vi "CSMinfo.vi"(4 "Error In":errorcluster, 7 "Command":string) -> (0 "Error Out":errorcluster, 3 "Response":string)   [LabVIEW 2018]
uses:
  MOKO_LabViewLibrary/MokoLowLevel/MokoLowLovelControl/MLLC_Mode.ctl
  data/CSMinfo.ctl
panel:
  in  "Utility name":string="CSMinfo"
  in  "Error Code":i32=5475
  in  "Settings":T2={"Saved Data"=variant, "Permanent data"={"Общие сведения"={"Регистрационный номер заказа"="", "Идентификация (шифр) образца"="", "IMEI образца"="", "НД, устанавливающий требования"="", "Методы испытаний (измерений)"="", "Дата начала испытаний"="", "Дата завершения испытаний"=""}, "Климатические условия внешней среды"={"Температура окружающего воздуха"="", "Относительная влажность воздуха"="", "Атмосферное давление"=""}, "Окно с настройками"={"Режим звонка связь"=0, "Напряжение источника"=0, "Условия окружающей среды"=0, "Номер образца"=0, "Источник питания"=0, "Номер испытания"=0, "Режим звонка тональный модем"=0, "Количество итераций TM"=100.0, "Аутентификация"=0, "Колличество повторов измерений"=1.0, "Сим карта"=0, "VISA adress of CMW500"="", "Input attenuation"=1.0, "Output attenuation"=1.0, "Call Release Type"=0, "GSM Band"=0, "BCCH Channel Number"=0.0, "TCH Channel Number"=0.0, "Codec"=0, "AWGN"=0, "snrRatioInDb"=0.0, "GSM Fading"=0, "UL C/I ratio"=0, "Use a custom network ID"=FALSE, "MCC (Mobile Country Code)"=0.0, "MNC (Mobile Network Code)"=0.0, "NCC (Network Color Code)"=0.0, "MNC digit count"=0, "BCC (Base station Color Code)"=0.0, "LAC (Location Area Code)"=0.0, "RAC (Routing Area Code)"=0.0, "Cell Identity"=0.0, "Override UE ID"=FALSE, "MCC (UE Mobile Country Code)"=0.0, "MNC (UE Mobile Network Code)"=0.0, "MSIN (Mobile Subscription ID)"=0.0, "InputScaleFactor"=0, "OutputScaleFactor"=0, "Post MSD wave file playback 3GPP  26.269 \nEU_DTMF_tones"=FALSE, "Scenario"=0, "AlAckBehavior"=0, "PSAP listens for PUSH"=FALSE, "BCCH Channel Power"=0.0, "TCH Channel Power"=0.0, "Setting Path"=path "", "Алгоритм дозвона"=0}}} {"Permanent data"."Окно с настройками"."Алгоритм дозвона" items=["Standart", "Recall"]; "Permanent data"."Окно с настройками"."AlAckBehavior" items=["POSITIVE", "CLEAR_DOWN", "LOOP_BACK_MSD_PART"]; "Permanent data"."Окно с настройками"."Scenario" items=["NORMAL", "NORMAL_IMMEDIATE_START", "TIMEOUT_T3", "ALLRV_REQ", "SUPPRESS_MSD", "SUPPRESS_ALACK", "SUPPRESS_SEND_MSD"]; "Permanent data"."Окно с настройками"."OutputScaleFactor" items=["ONE", "QUARTER", "HALF", "TWO", "FOUR"]; "Permanent data"."Окно с настройками"."InputScaleFactor" items=["ONE", "QUARTER", "HALF", "TWO", "FOUR"]; "Permanent data"."Окно с настройками"."MNC digit count" items=["TWO", "THREE"]; "Permanent data"."Окно с настройками"."UL C/I ratio" items=["Ci1Db", "Ci4Db", "Ci7Db", "Ci10Db", "Ci13Db", "Ci16Db"]; "Permanent data"."Окно с настройками"."GSM Fading" items=["GsmFadingOff", "GsmEtsiTs103412DlFading", "GsmEtsiTs103412UlFading", "GsmEtsiTs103412DlUlFading"]; "Permanent data"."Окно с настройками"."AWGN" items=["Off", "50MhzAwgn"]; "Permanent data"."Окно с настройками"."Codec" items=["FRV2", "AMRH_GMSK_7K95", "AMRH_GMSK_7K40", "AMRH_GMSK_6K70", "AMRH_GMSK_5K90", "AMRH_GMSK_5K15", "AMRH_GMSK_4K75", "AMRF_GMSK_12K20", "AMRF_GMSK_10K20", "AMRF_GMSK_7K95", "AMRF_GMSK_7K40 ", "AMRF_GMSK_6K70", "AMRF_GMSK_5K90", "AMRF_GMSK_5K15", "AMRF_GMSK_4K75", "FRV1", "HRV1", "WAMR_GMSK_6K60", "WAMR_GMSK_8K85", "WAMR_GMSK_12K65"]; "Permanent data"."Окно с настройками"."GSM Band" items=["GSM450", "GSM850", "GSM900", "GSM1800", "GSM1900"]; "Permanent data"."Окно с настройками"."Call Release Type" items=["NormalRelease", "CallInterruption"]; "Permanent data"."Окно с настройками"."Сим карта" items=["SIM", "eSIM"]; "Permanent data"."Окно с настройками"."Колличество повторов измерений" min=1.0 max=100.0 format="%#_3g"; "Permanent data"."Окно с настройками"."Аутентификация" items=["On", "Off"]; "Permanent data"."Окно с настройками"."Режим звонка тональный модем" items=["Автоматически (AT) GEMALTO", "Автоматически (AT) SIMCOM", "Автоматически (AT) SIMCOM SIM7600E-H", "Автоматически (AT) TELIT", "Автоматически (AT) PROGRESS", "Автоматически (AT) PROGRESS GREEN", "Автоматически (AT) PROGRESS BLUE", "Автоматически (реле)", "Вручную"]; "Permanent data"."Окно с настройками"."Номер испытания" items=["1", "2", "3"]; "Permanent data"."Окно с настройками"."Источник питания" items=["Не используется", "IT6332A"]; "Permanent data"."Окно с настройками"."Номер образца" items=["1", "2", "3"]; "Permanent data"."Окно с настройками"."Условия окружающей среды" items=["UnormTnorm", "UminTmin", "UmaxTmin", "UminTmax", "UmaxTmax", "TypeA", "TypeB"]; "Permanent data"."Окно с настройками"."Напряжение источника" items=["12", "24"]; "Permanent data"."Окно с настройками"."Режим звонка связь" items=["Автоматически (AT) GEMALTO", "Автоматически (AT) SIMCOM", "Автоматически (AT) SIMCOM SIM7600E-H", "Автоматически (AT) TELIT", "Автоматически (AT) PROGRESS", "Автоматически (AT) PROGRESS GREEN", "Автоматически (AT) PROGRESS BLUE", "Автоматически (реле)", "Вручную"]}
  in  "Mode":T3=enum."Check"
  # "CSMinfo"
  # "Default Settings"
  # "1. Общие настройки"
  # "Настройки модема по умолчанию"
  # "CMW500"
  # "PSAP"
  # "8.6.6"
  # "8.6.7"
  # "GSM"
  # "2. Настройки связи"
  # "8.6.8 (Use parameter NORMAL_IMMEDIATE_START)"
  # "8.6.9 (Use parameter LOOP_BACK_MSD_PART)"
  # "8.6.6"
  # "3. Настройки тонального модема"
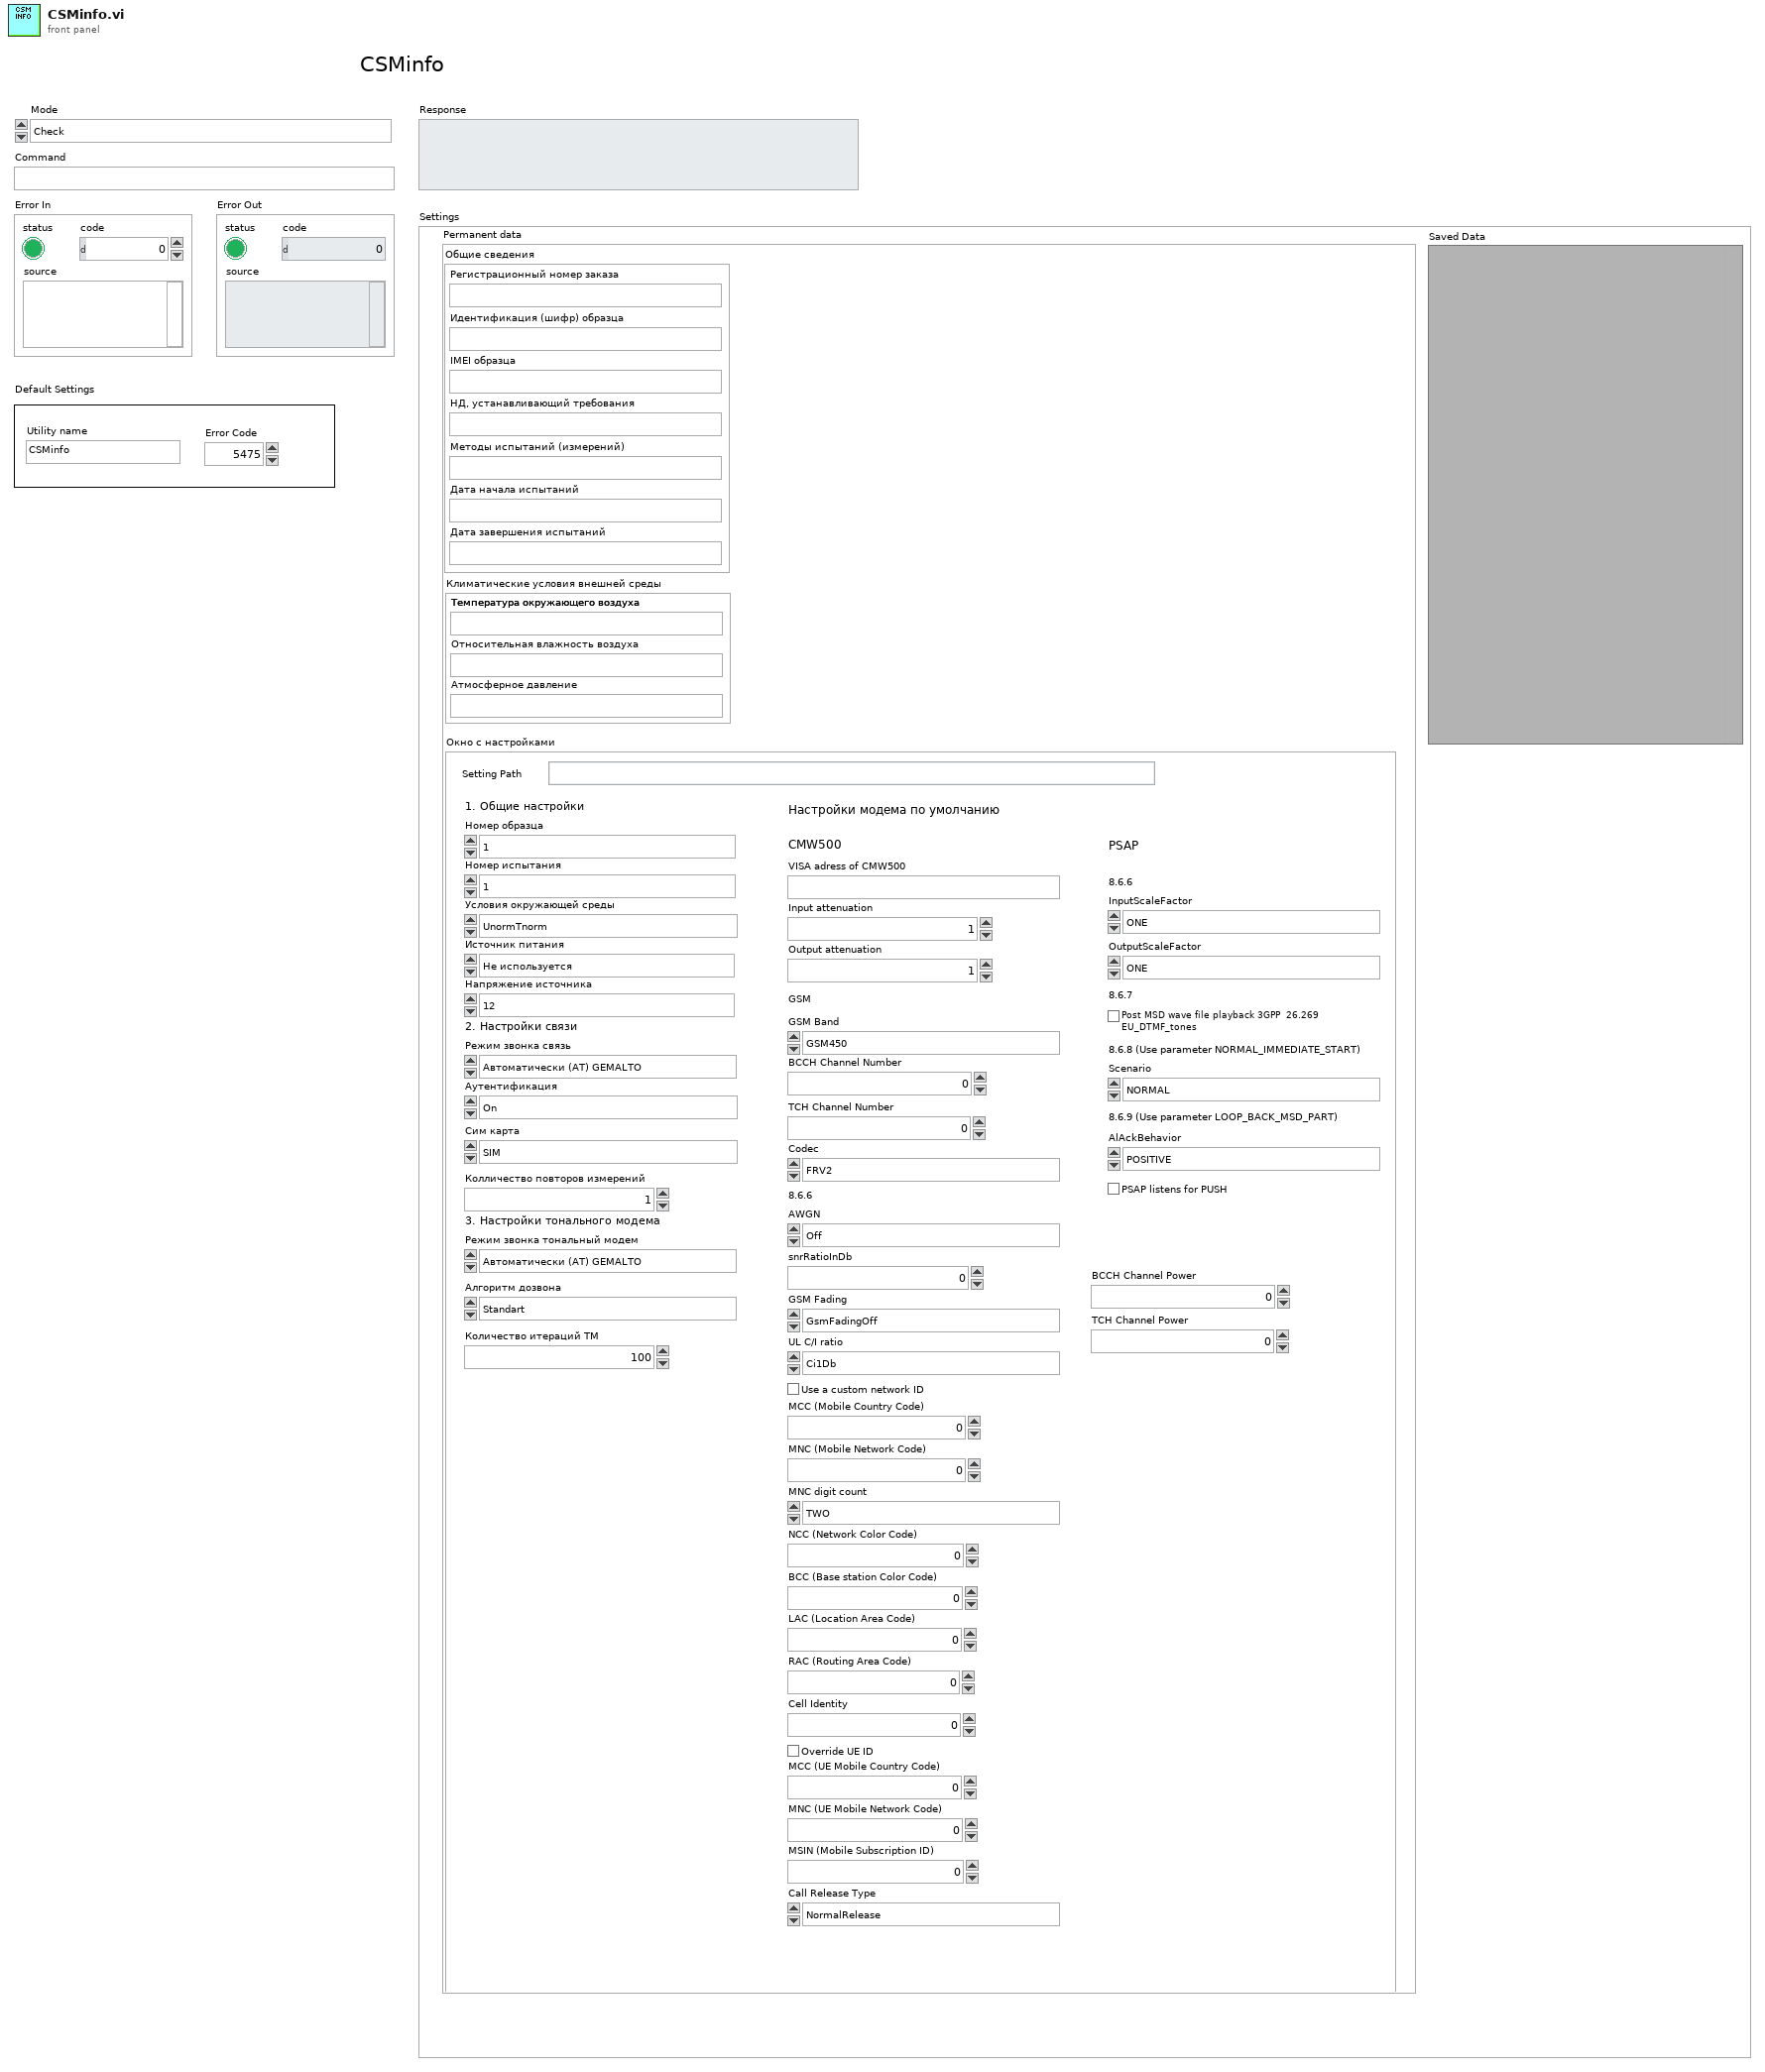
[diagram p1: front panel]
types:
  T1 = typedef "CSMinfo.ctl" = cluster{"Общие сведения":cluster{"Регистрационный номер заказа":string, "Идентификация (шифр) образца":string, "IMEI образца":string, "НД, устанавливающий требования":string, "Методы испытаний (измерений)":string, "Дата начала испытаний":string, "Дата завершения испытаний":string}, "Климатические условия внешней среды":cluster{"Температура окружающего воздуха":string, "Относительная влажность воздуха":string, "Атмосферное давление":string}, "Окно с настройками":cluster{"Режим звонка связь":u16, "Напряжение источника":u16, "Условия окружающей среды":u16, "Номер образца":u16, "Источник питания":u16, "Номер испытания":u16, "Режим звонка тональный модем":u16, "Количество итераций TM":dbl, "Аутентификация":u16, "Колличество повторов измерений":dbl, "Сим карта":u16, "VISA adress of CMW500":string, "Input attenuation":dbl, "Output attenuation":dbl, "Call Release Type":u16, "GSM Band":u16, "BCCH Channel Number":dbl, "TCH Channel Number":dbl, "Codec":u16, "AWGN":u16, "snrRatioInDb":dbl, "GSM Fading":u16, "UL C/I ratio":u16, "Use a custom network ID":bool, "MCC (Mobile Country Code)":dbl, "MNC (Mobile Network Code)":dbl, "NCC (Network Color Code)":dbl, "MNC digit count":u16, "BCC (Base station Color Code)":dbl, "LAC (Location Area Code)":dbl, "RAC (Routing Area Code)":dbl, "Cell Identity":dbl, "Override UE ID":bool, "MCC (UE Mobile Country Code)":dbl, "MNC (UE Mobile Network Code)":dbl, "MSIN (Mobile Subscription ID)":dbl, "InputScaleFactor":u16, "OutputScaleFactor":u16, "Post MSD wave file playback 3GPP  26.269 \nEU_DTMF_tones":bool, "Scenario":u16, "AlAckBehavior":u16, "PSAP listens for PUSH":bool, "BCCH Channel Power":dbl, "TCH Channel Power":dbl, "Setting Path":path, "Алгоритм дозвона":u16}}
  T2 = cluster{"Saved Data":variant, "Permanent data":T1}
  T3 = typedef "MLLC_Mode.ctl" = enum16{"get", "set", "close", "Init", "Check"}
  T4 = typedef "MLLC_Error.ctl" = errorcluster
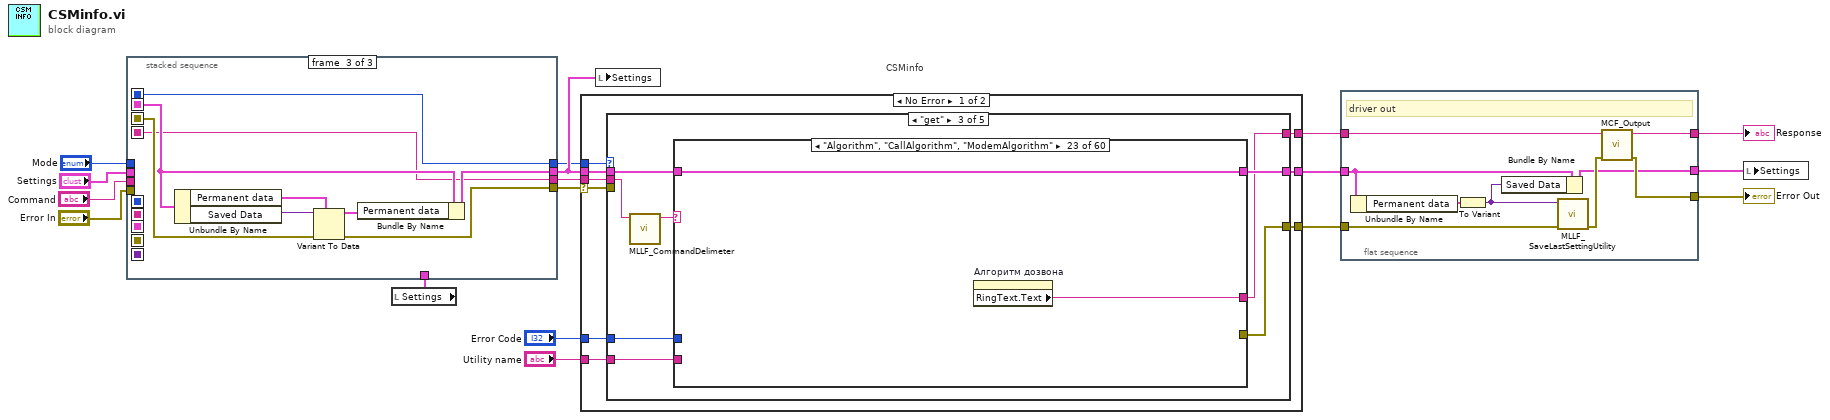
[diagram p0: block diagram]
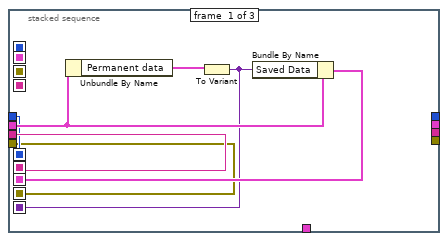
[diagram p2: hidden frame]
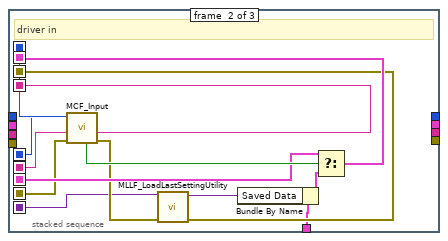
[diagram p3: hidden frame]
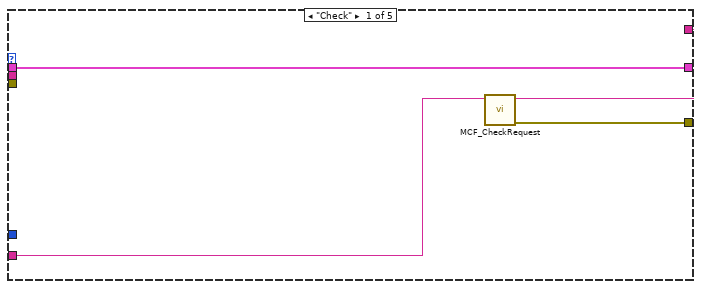
[diagram p4: hidden frame]
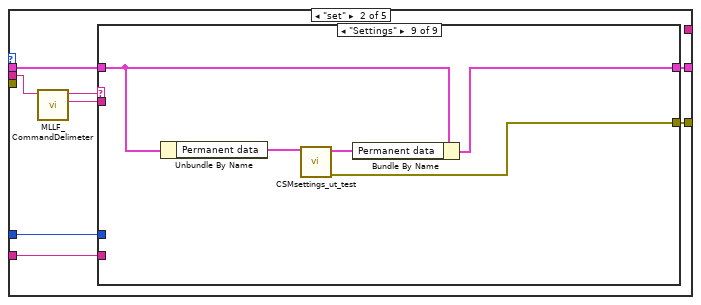
[diagram p5: hidden frame]
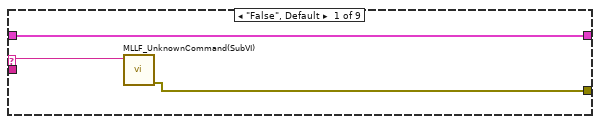
[diagram p6: hidden frame]
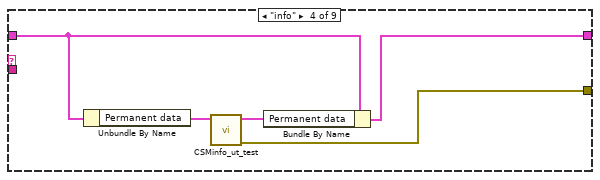
[diagram p9: hidden frame]
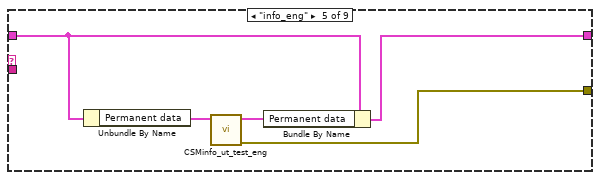
[diagram p10: hidden frame]
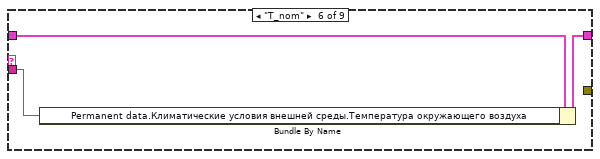
[diagram p11: hidden frame]
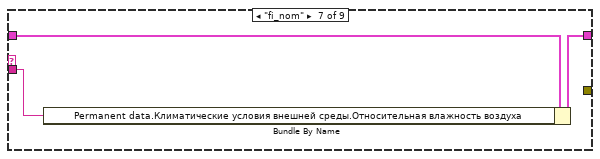
[diagram p12: hidden frame]
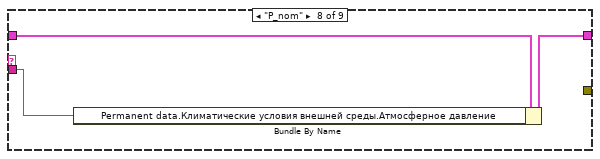
[diagram p13: hidden frame]
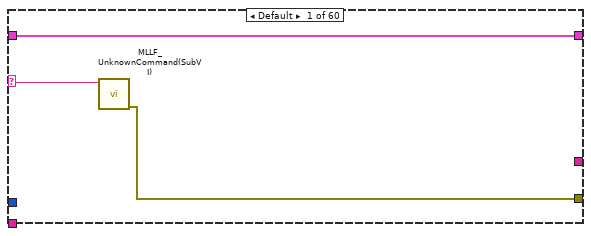
[diagram p14: hidden frame]
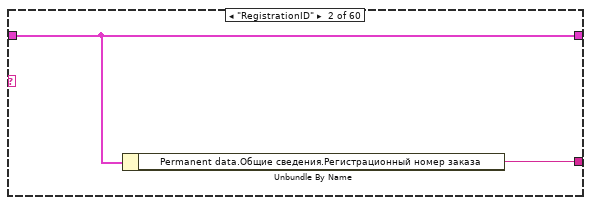
[diagram p15: hidden frame]
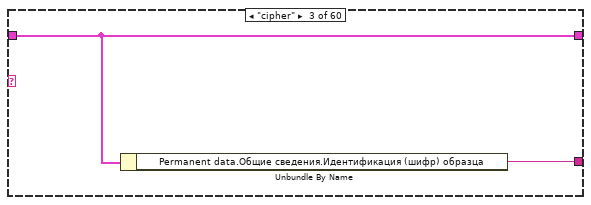
[diagram p16: hidden frame]
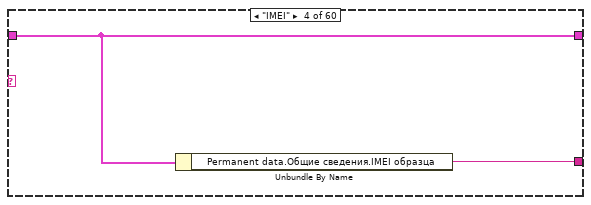
[diagram p17: hidden frame]
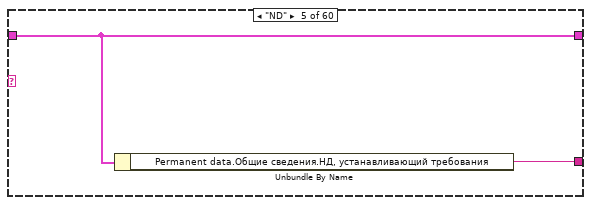
[diagram p18: hidden frame]
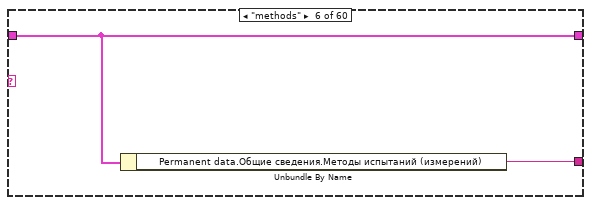
[diagram p19: hidden frame]
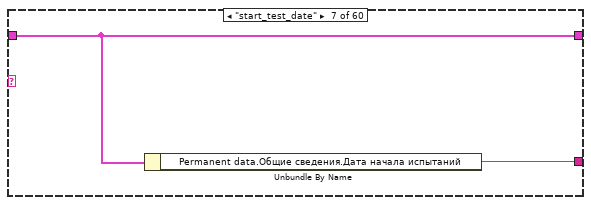
[diagram p20: hidden frame]
diagram:
  # "CSMinfo"
  n1 = local read "Settings"() -> (w12:T2)
  n2 = stacked-sequence {
    seq-local: [w20 _ _] -> [_ w36 _]
    seq-local: [w19 _ _] -> [_ w37 _]
    seq-local: [w22 _ _] -> [_ w32 _]
    seq-local: [w18 _ _] -> [_ w31 _]
    seq-local: [w21 _ _] -> [_ w26 _]
    seq-local: [_ w27 _] -> [_ _ w43]
    seq-local: [_ w38 _] -> [_ _ w40]
    seq-local: [_ w35 _] -> [_ _ w39]
    seq-local: [_ w34 _] -> [_ _ w44]
    tunnel: "Command" -> [w20 _ _]
    tunnel: "Mode" -> [w19 _ _]
    tunnel: "Error In" -> [w18 _ _]
    tunnel: "Settings" -> [w23 _ _]
    tunnel: w12 -> [_ w25 _]
    tunnel: [_ _ w39] -> w8
    tunnel: [_ _ w42] -> w11
    tunnel: [_ _ w41] -> w10
    tunnel: [_ _ w40] -> w9
    frame #0 {
      n3 = Unbundle By Name(w23) -> ("Permanent data"=w24:T1)
      n4 = To Variant(anything=w24) -> (Variant=w21:variant)
      n5 = Bundle By Name(cluster=w23, "Saved Data"=w21) -> (w22:T2)
    }
    frame #1 {
      # "driver in"
      n6 = call "MCF_Input.vi"("Error In"=w31, "Command in"=w36, "Mode in"=w37) -> ("Error Out"=w30:errorcluster, "Command out"=w35:string, "Mode out"=w38:T3, "Boolean"=w33:bool)  [unwired: 5 in]
      n7 = call "MLLF_LoadLastSettingUtility.vi"("Error In"=w30, "Save data in"=w26) -> ("Error Out"=w27:errorcluster, "Save data out"=w29:variant)  [unwired: 8 in]
      n8 = Bundle By Name(cluster=w25, "Saved Data"=w29) -> (w28:T2)
      n9 = Select(t=w32, s=w33, f=w28) -> (s? t:f=w34:T2)
    }
    frame #2 {
      n10 = Unbundle By Name(w44) -> ("Permanent data"=w45:T1, "Saved Data"=w47:variant)
      n11 = Variant To Data(error in=w43, type=w45, Variant=w47) -> (data=w46:T1, error out=w41:errorcluster)
      n12 = Bundle By Name(cluster=w44, "Permanent data"=w46) -> (w42:T2)
    }
  }
  n13 = case shown="No Error" w10 {
    selector: w10 -> [w52 w238]
    tunnel: [w54 w238] -> w16
    tunnel: w9 -> [w56 _]
    tunnel: [w55 _] -> w14
    tunnel: w8 -> [w53 _]
    tunnel: w11 -> [w49 w237]
    tunnel: "Error Code" -> [w51 _]
    tunnel: "Utility name" -> [w50 _]
    tunnel: [w48 w237] -> w15
    frame No Error {
      n14 = case shown="\"get\"" w56 {
        tunnel: [w58 _ w99 _ _] -> w55
        tunnel: [w57 w67 w98 _ _] -> w54
        tunnel: w53 -> [_ w68 w105 _ _]
        tunnel: w52 -> [_ _ _ _ _]
        tunnel: w51 -> [_ w66 w103 _ _]
        tunnel: w50 -> [w59 w63 w102 _ _]
        tunnel: w49 -> [w60 w65 w104 w235 w236]
        tunnel: [w60 w64 w101 w235 w236] -> w48
        frame "Check" {
          n15 = call "MCF_CheckRequest.vi"("Driver Name"=w59) -> ("Error Out"=w57:errorcluster, "Output String"=w58:string)  [unwired: 9 in]
        }
        frame "set" {
          n16 = call "MLLF_CommandDelimeter.vi"("command with param"=w68) -> ("param 1"=w61:string, "command"=w62:string)  [unwired: 6 in, 3 out]
          n17 = case shown="\"Settings\"" w62 {
            selector: w62 -> [w70 _ _ _ _ _ _ _ _]
            tunnel: w61 -> [_ _ _ _ _ w84 w87 w90 _]
            tunnel: [w69 _ _ w78 w83 _ _ _ w97] -> w67
            tunnel: w66 -> [_ _ _ _ _ _ _ _ _]
            tunnel: w65 -> [w71 w72 w73 w77 w82 w86 w89 w92 w95]
            tunnel: [w71 w72 w73 w76 w81 w85 w88 w91 w96] -> w64
            tunnel: w63 -> [_ _ _ _ _ _ _ _ _]
            frame "False", Default {
              n18 = call "MLLF_UnknownCommand(SubVI).vi"("Unknown command"=w70) -> ("error out"=w69:errorcluster)  [unwired: 10 in]
            }
            frame "<----MAIN FUNCTIONS---->" {
            }
            frame "---------ADDITIONAL---------" {
            }
            frame "info" {
              n19 = Unbundle By Name(w77) -> ("Permanent data"=w74:T1)
              n20 = call "CSMinfo_ut_test.vi"("CSMinfo in"=w74) -> ("Error Out"=w78:errorcluster, "CSMinfo out"=w75:T1)  [unwired: 9 in]
              n21 = Bundle By Name(cluster=w77, "Permanent data"=w75) -> (w76:T2)
            }
            frame "info_eng" {
              n22 = Unbundle By Name(w82) -> ("Permanent data"=w79:T1)
              n23 = call "CSMinfo_ut_test_eng.vi"("CSMinfo in"=w79) -> ("Error Out"=w83:errorcluster, "CSMinfo out"=w80:T1)  [unwired: 9 in]
              n24 = Bundle By Name(cluster=w82, "Permanent data"=w80) -> (w81:T2)
            }
            frame "T_nom" {
              n25 = Bundle By Name(cluster=w86, "Permanent data.Климатические условия внешней среды.Температура окружающего воздуха"=w84) -> (w85:T2)
            }
            frame "fi_nom" {
              n26 = Bundle By Name(cluster=w89, "Permanent data.Климатические условия внешней среды.Относительная влажность воздуха"=w87) -> (w88:T2)
            }
            frame "P_nom" {
              n27 = Bundle By Name(cluster=w92, "Permanent data.Климатические условия внешней среды.Атмосферное давление"=w90) -> (w91:T2)
            }
            frame "Settings" {
              n28 = Unbundle By Name(w95) -> ("Permanent data"=w94:T1)
              n29 = call "CSMsettings_ut_test.vi"("CSMinfo in"=w94) -> ("Error Out"=w97:errorcluster, "CSMinfo out"=w93:T1)  [unwired: 9 in]
              n30 = Bundle By Name(cluster=w95, "Permanent data"=w93) -> (w96:T2)
            }
          }
        }
        frame "get" {
          n31 = call "MLLF_CommandDelimeter.vi"("command with param"=w105) -> ("command"=w100:string)  [unwired: 6 in, 4 out]
          n32 = case shown="\"Algorithm\", \"CallAlgorithm\", \"ModemAlgorithm\"" w100 {
            selector: w100 -> [w107 _ _ _ _ _ _ _ _ _ _ _ _ _ _ _ _ _ _ _ _ _ _ _ _ _ _ _ _ _ _ _ _ _ _ _ _ _ _ _ _ _ _ _ _ _ _ _ _ _ _ _ _ _ _ _ _ _ _ _]
            tunnel: [w106 _ _ _ _ _ _ _ _ _ _ _ _ _ _ _ _ _ _ _ _ _ _ _ _ _ _ _ _ _ _ _ _ _ _ _ _ _ _ _ _ _ _ _ _ _ _ _ _ _ _ _ _ _ _ _ _ _ _ _] -> w98
            tunnel: w103 -> [_ _ _ _ _ _ _ _ _ _ _ _ _ _ _ _ _ _ _ _ _ _ _ _ _ _ _ _ _ _ _ _ _ _ _ _ _ _ _ _ _ _ _ _ _ _ _ _ _ _ _ _ _ _ _ _ _ _ _ _]
            tunnel: [w108 w109 w111 w113 w115 w117 w119 w121 w123 w125 w127 w129 w131 w133 w135 w137 w139 w141 w143 w145 w147 w149 w151 w153 w154 w156 w158 w160 w161 w163 w165 w167 w169 w170 w172 w174 w177 w179 w181 w186 w188 w190 w192 w194 w196 w198 w200 w202 w207 w209 w211 w213 w215 w216 w218 w220 w225 w227 w229 w234] -> w101
            tunnel: w104 -> [w108 w109 w111 w113 w115 w117 w119 w121 w123 w125 w127 w129 w131 w133 w135 w137 w139 w141 w143 w145 w147 w149 w151 w153 w154 w156 w158 w160 w161 w163 w165 w167 w169 w170 w172 w174 w177 w179 w181 w186 w188 w190 w192 w194 w196 w198 w200 w202 w207 w209 w211 w213 w215 w216 w218 w220 w225 w227 w229 w234]
            tunnel: w102 -> [_ _ _ _ _ _ _ _ _ _ _ _ _ _ _ _ _ _ _ _ _ _ _ _ _ _ _ _ _ _ _ _ _ _ _ _ _ _ _ _ _ _ _ _ _ _ _ _ _ _ _ _ _ _ _ _ _ _ _ _]
            tunnel: [_ w110 w112 w114 w116 w118 w120 w122 w124 w126 w128 _ w130 w132 w134 w136 w138 w140 w142 w144 w146 w148 w150 w152 _ w155 w157 w159 _ w162 w164 w166 w168 w171 w173 w175 w176 w178 w180 w182 w187 w189 w191 w193 w195 w197 w199 w201 w203 w208 w210 w212 w214 _ w217 w219 w221 w226 w228 w230] -> w99
            frame Default {
              n33 = call "MLLF_UnknownCommand(SubVI).vi"("Unknown command"=w107) -> ("error out"=w106:errorcluster)  [unwired: 10 in]
            }
            frame "RegistrationID" {
              n34 = Unbundle By Name(w109) -> ("Permanent data.Общие сведения.Регистрационный номер заказа"=w110:string)
            }
            frame "cipher" {
              n35 = Unbundle By Name(w111) -> ("Permanent data.Общие сведения.Идентификация (шифр) образца"=w112:string)
            }
            frame "IMEI" {
              n36 = Unbundle By Name(w113) -> ("Permanent data.Общие сведения.IMEI образца"=w114:string)
            }
            frame "ND" {
              n37 = Unbundle By Name(w115) -> ("Permanent data.Общие сведения.НД, устанавливающий требования"=w116:string)
            }
            frame "methods" {
              n38 = Unbundle By Name(w117) -> ("Permanent data.Общие сведения.Методы испытаний (измерений)"=w118:string)
            }
            frame "start_test_date" {
              n39 = Unbundle By Name(w119) -> ("Permanent data.Общие сведения.Дата начала испытаний"=w120:string)
            }
            frame "completion_test_date" {
              n40 = Unbundle By Name(w121) -> ("Permanent data.Общие сведения.Дата завершения испытаний"=w122:string)
            }
            frame "T_nom" {
              n41 = Unbundle By Name(w123) -> ("Permanent data.Климатические условия внешней среды.Температура окружающего воздуха"=w124:string)
            }
            frame "fi_nom" {
              n42 = Unbundle By Name(w125) -> ("Permanent data.Климатические условия внешней среды.Относительная влажность воздуха"=w126:string)
            }
            frame "P_nom" {
              n43 = Unbundle By Name(w127) -> ("Permanent data.Климатические условия внешней среды.Атмосферное давление"=w128:string)
            }
            frame "------------------- SETTINGS -----------------" {
            }
            frame "SampleNumber" {
              n44 = property on="Номер образца" class="Ring (strict)"() -> ("RingText.Text"=w130:string)  [unwired: 2 in, 2 out]
            }
            frame "TestNumber" {
              n45 = property on="Номер испытания" class="Ring (strict)"() -> ("RingText.Text"=w132:string)  [unwired: 2 in, 2 out]
            }
            frame "EnvironmentalConditions" {
              n46 = property on="Условия окружающей среды" class="Ring (strict)"() -> ("RingText.Text"=w134:string)  [unwired: 2 in, 2 out]
            }
            frame "PowerSupply" {
              n47 = property on="Источник питания" class="Ring (strict)"() -> ("RingText.Text"=w136:string)  [unwired: 2 in, 2 out]
            }
            frame "SourceVoltage" {
              n48 = property on="Напряжение источника" class="Ring (strict)"() -> ("RingText.Text"=w138:string)  [unwired: 2 in, 2 out]
            }
            frame "CallModeSignal" {
              n49 = property on="Режим звонка связь" class="Ring (strict)"() -> ("RingText.Text"=w140:string)  [unwired: 2 in, 2 out]
            }
            frame "authentication" {
              n50 = property on="Аутентификация" class="Ring (strict)"() -> ("RingText.Text"=w142:string)  [unwired: 2 in, 2 out]
            }
            frame "SimCard" {
              n51 = property on="Сим карта" class="Ring (strict)"() -> ("RingText.Text"=w144:string)  [unwired: 2 in, 2 out]
            }
            frame "NumberOfMeasurements" {
              n52 = property on="Колличество повторов измерений" class="DigNum (strict)"() -> ("NumText.Text"=w146:string)  [unwired: 2 in, 2 out]
            }
            frame "CallModeToneModem" {
              n53 = property on="Режим звонка тональный модем" class="Ring (strict)"() -> ("RingText.Text"=w148:string)  [unwired: 2 in, 2 out]
            }
            frame "Algorithm", "CallAlgorithm", "ModemAlgorithm" {
              n54 = property on="Алгоритм дозвона" class="Ring (strict)"() -> ("RingText.Text"=w150:string)  [unwired: 2 in, 2 out]
            }
            frame "ToneModemIterations" {
              n55 = property on="Количество итераций TM" class="DigNum (strict)"() -> ("NumText.Text"=w152:string)  [unwired: 2 in, 2 out]
            }
            frame "---------------- ВКЛАДКА CMW --------------" {
            }
            frame "adress", "VISA", "VISAadress" {
              n56 = property on="VISA adress of CMW500" class="Str"() -> ("Text.Text"=w155:string)  [unwired: 2 in, 2 out]
            }
            frame "InputAtt", "InputAttenuation" {
              n57 = property on="Input attenuation" class="DigNum (strict)"() -> ("NumText.Text"=w157:string)  [unwired: 2 in, 2 out]
            }
            frame "OutputAtt", "OutputAttenuation" {
              n58 = property on="Output attenuation" class="DigNum (strict)"() -> ("NumText.Text"=w159:string)  [unwired: 2 in, 2 out]
            }
            frame "---------------- ВКЛАДКА GSM --------------" {
            }
            frame "Band" {
              n59 = property on="GSM Band" class="Ring (strict)"() -> ("RingText.Text"=w162:string)  [unwired: 2 in, 2 out]
            }
            frame "bcchPower" {
              n60 = property on="BCCH Channel Power" class="DigNum (strict)"() -> ("NumText.Text"=w164:string)  [unwired: 2 in, 2 out]
            }
            frame "tchPower" {
              n61 = property on="TCH Channel Power" class="DigNum (strict)"() -> ("NumText.Text"=w166:string)  [unwired: 2 in, 2 out]
            }
            frame "bcchNum" {
              n62 = property on="BCCH Channel Number" class="DigNum (strict)"() -> ("NumText.Text"=w168:string)  [unwired: 2 in, 2 out]
            }
            frame "tchNum" {
              n63 = property on="TCH Channel Number" class="DigNum (strict)"() -> ("NumText.Text"=w171:string)  [unwired: 2 in, 2 out]
            }
            frame "Codec" {
              n64 = property on="Codec" class="Ring (strict)"() -> ("RingText.Text"=w173:string)  [unwired: 2 in, 2 out]
            }
            frame "AWGN" {
              n65 = property on="AWGN" class="Ring (strict)"() -> ("RingText.Text"=w175:string)  [unwired: 2 in, 2 out]
            }
            frame "snrRatio", "snrRatioInDb" {
              n66 = property on="snrRatioInDb" class="DigNum (strict)"() -> ("NumText.Text"=w176:string)  [unwired: 2 in, 2 out]
            }
            frame "GsmFading" {
              n67 = property on="GSM Fading" class="Ring (strict)"() -> ("RingText.Text"=w178:string)  [unwired: 2 in, 2 out]
            }
            frame "GsmFadingCI" {
              n68 = property on="UL C/I ratio" class="Ring (strict)"() -> ("RingText.Text"=w180:string)  [unwired: 2 in, 2 out]
            }
            frame "customNetworkID" {
              n69 = property on="Use a custom network ID" class="Bool (strict)"() -> ("Value"=w185:bool)  [unwired: 2 in, 2 out]
              n70 = Select(t="true", s=w185, f="false") -> (s? t:f=w182:string)
            }
            frame "MCC" {
              n71 = property on="MCC (Mobile Country Code)" class="DigNum (strict)"() -> ("NumText.Text"=w187:string)  [unwired: 2 in, 2 out]
            }
            frame "MNC" {
              n72 = property on="MNC (Mobile Network Code)" class="DigNum (strict)"() -> ("NumText.Text"=w189:string)  [unwired: 2 in, 2 out]
            }
            frame "mncMode" {
              n73 = property on="MNC digit count" class="Ring (strict)"() -> ("RingText.Text"=w191:string)  [unwired: 2 in, 2 out]
            }
            frame "NCC" {
              n74 = property on="NCC (Network Color Code)" class="DigNum (strict)"() -> ("NumText.Text"=w193:string)  [unwired: 2 in, 2 out]
            }
            frame "BCC" {
              n75 = property on="BCC (Base station Color Code)" class="DigNum (strict)"() -> ("NumText.Text"=w195:string)  [unwired: 2 in, 2 out]
            }
            frame "LAC" {
              n76 = property on="LAC (Location Area Code)" class="DigNum (strict)"() -> ("NumText.Text"=w197:string)  [unwired: 2 in, 2 out]
            }
            frame "RAC" {
              n77 = property on="RAC (Routing Area Code)" class="DigNum (strict)"() -> ("NumText.Text"=w199:string)  [unwired: 2 in, 2 out]
            }
            frame "CID" {
              n78 = property on="Cell Identity" class="DigNum (strict)"() -> ("NumText.Text"=w201:string)  [unwired: 2 in, 2 out]
            }
            frame "customUEID" {
              n79 = property on="Override UE ID" class="Bool (strict)"() -> ("Value"=w206:bool)  [unwired: 2 in, 2 out]
              n80 = Select(t="true", s=w206, f="false") -> (s? t:f=w203:string)
            }
            frame "UEMCC" {
              n81 = property on="MCC (UE Mobile Country Code)" class="DigNum (strict)"() -> ("NumText.Text"=w208:string)  [unwired: 2 in, 2 out]
            }
            frame "UEMNC" {
              n82 = property on="MNC (UE Mobile Network Code)" class="DigNum (strict)"() -> ("NumText.Text"=w210:string)  [unwired: 2 in, 2 out]
            }
            frame "UEMSIN" {
              n83 = property on="MSIN (Mobile Subscription ID)" class="DigNum (strict)"() -> ("NumText.Text"=w212:string)  [unwired: 2 in, 2 out]
            }
            frame "CallReleaseType" {
              n84 = property on="Call Release Type" class="Ring (strict)"() -> ("RingText.Text"=w214:string)  [unwired: 2 in, 2 out]
            }
            frame "-------------------- PSAP -------------------" {
            }
            frame "inputScaleFactor" {
              n85 = property on="InputScaleFactor" class="Ring (strict)"() -> ("RingText.Text"=w217:string)  [unwired: 2 in, 2 out]
            }
            frame "outputScaleFactor" {
              n86 = property on="OutputScaleFactor" class="Ring (strict)"() -> ("RingText.Text"=w219:string)  [unwired: 2 in, 2 out]
            }
            frame "PostMSDwavefileplayback" {
              n87 = property on="Post MSD wave file playback 3GPP  26.269 \nEU_DTMF_tones" class="Bool (strict)"() -> ("Value"=w224:bool)  [unwired: 2 in, 2 out]
              n88 = Select(t="true", s=w224, f="false") -> (s? t:f=w221:string)
            }
            frame "Scenario" {
              n89 = property on="Scenario" class="Ring (strict)"() -> ("RingText.Text"=w226:string)  [unwired: 2 in, 2 out]
            }
            frame "AlAckBehavior" {
              n90 = property on="AlAckBehavior" class="Ring (strict)"() -> ("RingText.Text"=w228:string)  [unwired: 2 in, 2 out]
            }
            frame "AudiobehavioroncallbackbyPSAP" {
              n91 = property on="PSAP listens for PUSH" class="Bool (strict)"() -> ("Value"=w233:bool)  [unwired: 2 in, 2 out]
              n92 = Select(t="true", s=w233, f="false") -> (s? t:f=w230:string)
            }
          }
        }
        frame "close" {
        }
        frame "Init" {
        }
      }
    }
    frame Error {
    }
  }
  n93 = local write "Settings"(w11) -> ()
  n94 = flat-sequence {
    tunnel: [w247] -> w6
    tunnel: [w246] -> w4
    tunnel: w14 -> [w245]
    tunnel: w16 -> [w244]
    tunnel: w15 -> [w240]
    tunnel: [w242] -> w13
    frame #0 {
      # "driver out"
      n95 = Unbundle By Name(w240) -> ("Permanent data"=w239:T1)
      n96 = To Variant(anything=w239) -> (Variant=w241:variant)
      n97 = Bundle By Name(cluster=w240, "Saved Data"=w241) -> (w242:T2)
      n98 = call "MLLF_SaveLastSettingUtility.vi"("error in"=w244, "Saved Data"=w241) -> ("error out"=w243:T4)  [unwired: 8 in, 1 out]
      n99 = call "MCF_Output.vi"("Error In"=w243, "Input"=w245) -> ("Error Out"=w246:errorcluster, "Output"=w247:string)  [unwired: 8 in]
    }
  }
  n100 = local write "Settings"(w13) -> ()
  "Response" <- w6
  "Error Out" <- w4
